vi "OxITC503 _Config_ Program One Sweep Stage.vi"(2 "Setpoint for Stage":dbl format="%.2f", 3 "Sweep Stage":i32=1 min=1 max=16 step=1, 4 "error in (no error)":errorcluster, 5 "Hold Time For Stage":dbl min=0.0 max=1339.9 step=0.1 format="%.2f", 6 "Sweep Time for Stage":dbl min=0.0 max=1339.9 step=0.1 format="%.2f", 7 "VISA session":refnum<visa-resource-name>) -> (0 "error out":errorcluster, 1 "VISA session":refnum<visa-resource-name>)   [LabVIEW 2013]
doc: "Allows programming the individual steps of the sweep table. Programmes the three y parameters ( set point temperature, sweep time to set point, hold time at set point) for a single step (between 1 to 16).\n\nITC503 must be in REMOTE mode and sweep must be not running."
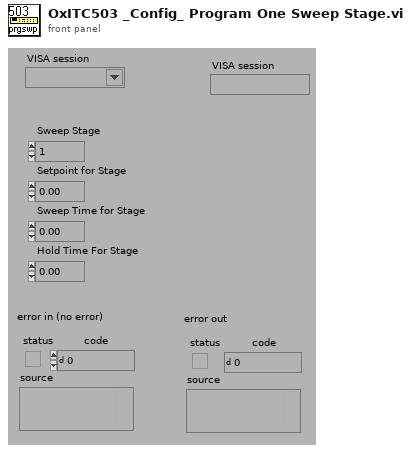
[diagram p1: front panel]
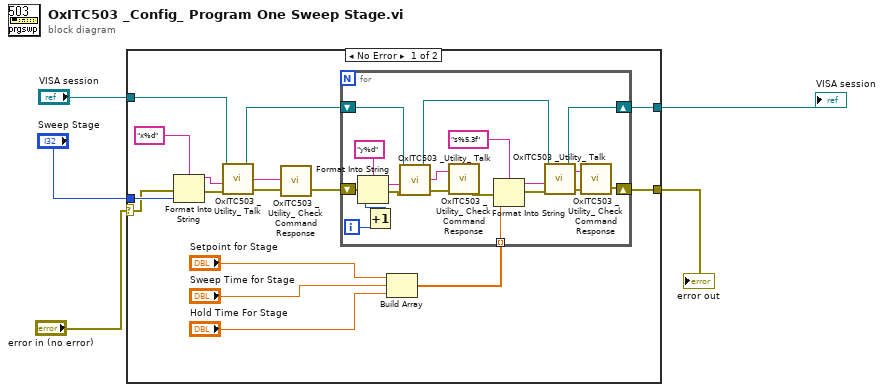
[diagram p0: block diagram]
diagram:
  n1 = case shown="No Error" "error in (no error)" {
    selector: "error in (no error)" -> [w6 w42]
    tunnel: "VISA session" -> [w21 w41]
    tunnel: "Sweep Stage" -> [w19 _]
    tunnel: [w8 w42] -> w3
    tunnel: [w7 w41] -> w2
    frame No Error {
      n2 = Format Into String(format string="x%d" ("Format String"), error in=w6, w19) -> (resulting string=w18:string, error out=w15:errorcluster)  [unwired: 1 in]
      n3 = call "OxITC503 _Utility_ Talk.vi"("VISA session"=w21, "Command"=w18, "error in (no error)"=w15) -> ("VISA session"=w10:refnum<visa-resource-name>, "read buffer"=w17:string, "error out (no error)"=w16:errorcluster)  [unwired: 2 in]
      n4 = call "OxITC503 _Utility_ Check Command Response.vi"("error in"=w16, "read buffer"=w17) -> ("error out (no error)"=w9:errorcluster)  [unwired: 1 out]
      n5 = Build Array("Setpoint for Stage", "Sweep Time for Stage", "Hold Time For Stage") -> (w11:dbl[])
      n6 = for {
        tunnel: w11 -> [w33] mode=indexing
        shift-right: [w31] -> w7
        shift-left: w10 -> [w32]
        shift-right: [w26] -> w8
        shift-left: w9 -> [w29]
        i -> [w30]
        n7 = Increment(x=w30) -> (x+1=w22:i32)
        n8 = Format Into String(format string="y%d" ("Format String"), error in=w29, w22) -> (resulting string=w23:string, error out=w28:errorcluster)  [unwired: 1 in]
        n9 = call "OxITC503 _Utility_ Talk.vi"("VISA session"=w32, "Command"=w23, "error in (no error)"=w28) -> ("VISA session"=w34:refnum<visa-resource-name>, "read buffer"=w39:string, "error out (no error)"=w40:errorcluster)  [unwired: 2 in]
        n10 = call "OxITC503 _Utility_ Check Command Response.vi"("error in"=w40, "read buffer"=w39) -> ("error out (no error)"=w38:errorcluster)  [unwired: 1 out]
        n11 = Format Into String(format string="s%5.3f" ("Format String"), error in=w38, w33) -> (resulting string=w35:string, error out=w36:errorcluster)  [unwired: 1 in]
        n12 = call "OxITC503 _Utility_ Talk.vi"("VISA session"=w34, "Command"=w35, "error in (no error)"=w36) -> ("VISA session"=w31:refnum<visa-resource-name>, "read buffer"=w25:string, "error out (no error)"=w27:errorcluster)  [unwired: 2 in]
        n13 = call "OxITC503 _Utility_ Check Command Response.vi"("error in"=w27, "read buffer"=w25) -> ("error out (no error)"=w26:errorcluster)  [unwired: 1 out]
      }
    }
    frame Error {
    }
  }
  "VISA session" <- w2
  "error out" <- w3
